vi "modify assembly.vi"(8 "error in":errorcluster, 9 "new":T1={"name"="", "Instance ID"=100, "Type"=enum."Producing", "Size (elements)"=32, "big endian?"=FALSE, "data type"=enum."Double"}, 10 "original":T1={"name"="", "Instance ID"=100, "Type"=enum."Producing", "Size (elements)"=32, "big endian?"=FALSE, "data type"=enum."Double"}, 11 "EthernetIP configuration in":refnum<class "EthernetIP configuration.lvclass">) -> (0 "error out":errorcluster, 1 "channel type/dir changed":refnum<class "EthernetIP Channel.lvclass">[](array[class]), 2 "invalidated channels":refnum<class "EthernetIP Channel.lvclass">[](array[class]), 3 "EthernetIP configuration out":refnum<class "EthernetIP configuration.lvclass">)   [LabVIEW 2013, in "EthernetIP configuration.lvclass"]
uses:
  EthernetIP configuration.lvclass
  assembly definition.ctl
  assembly type.ctl
  <vilib>/NI/Tag Bus/tag/Data Type.ctl
  channel/EthernetIP Channel.lvclass
  EthernetIP configuration.lvclass/EthernetIP configuration.ctl
  channel/EthernetIP Channel.lvclass/EthernetIP Channel.ctl
  <vilib>/NI/Tag Bus Module Framework/channel/TBM channel.lvclass/TBM channel.ctl
  <vilib>/NI/Tag Bus/tag/tag descriptor.lvclass/tag descriptor.ctl
  channel/Write Instance ID.vi
  <vilib>/NI/Tag Bus Module Framework/channel/Read channel classification.vi
  <vilib>/NI/Tag Bus Module Framework/channel/Write channel classification.vi
  channel/Read byte index.vi
  <vilib>/NI/Tag Bus/tag/read data type.vi
  <vilib>/NI/Tag Bus/tag/write data type.vi
  <vilib>/NI/Tag Bus/tag/tag descriptor.lvclass
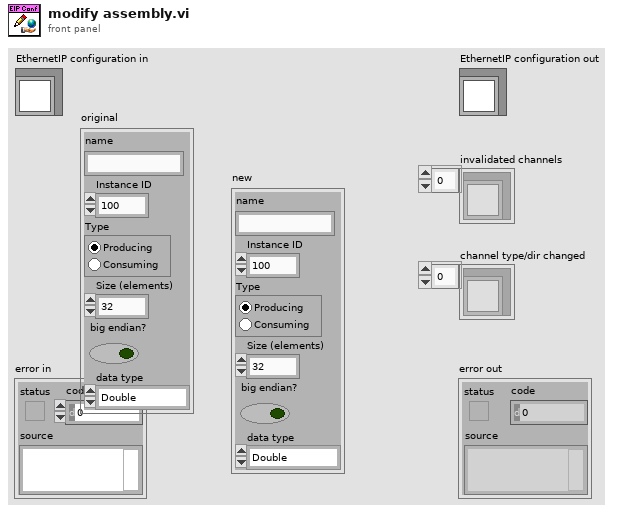
[diagram p1: front panel]
types:
  T1 = typedef "EthernetIP configuration.lvclass/assembly definition.ctl" = cluster{"name":string, "Instance ID":u32, "Type":T2, "Size (elements)":u32, "big endian?":bool, "data type":T3}
  T2 = typedef "EthernetIP configuration.lvclass/assembly type.ctl" = enum32{"Producing", "Consuming"}
  T3 = typedef "tag bus.lvlib/tag descriptor.lvclass/Data Type.ctl" = enum16{"Double", "Single", "I64", "I32", "I16", "I8", "U64", "U32", "U16", "U8", "Boolean", "String", "Array of Double", "Array of Single", "Array of I64", "Array of I32", "Array of I16", "Array of I8", "Array of U64", "Array of U32", "Array of U16", "Array of U8", "Array of Boolean", "Array of String"}
  T4 = typedef "TBM channel.lvclass/channel classification.ctl" = enum16{"input data", "output data", "processing parameter", "processing result"}
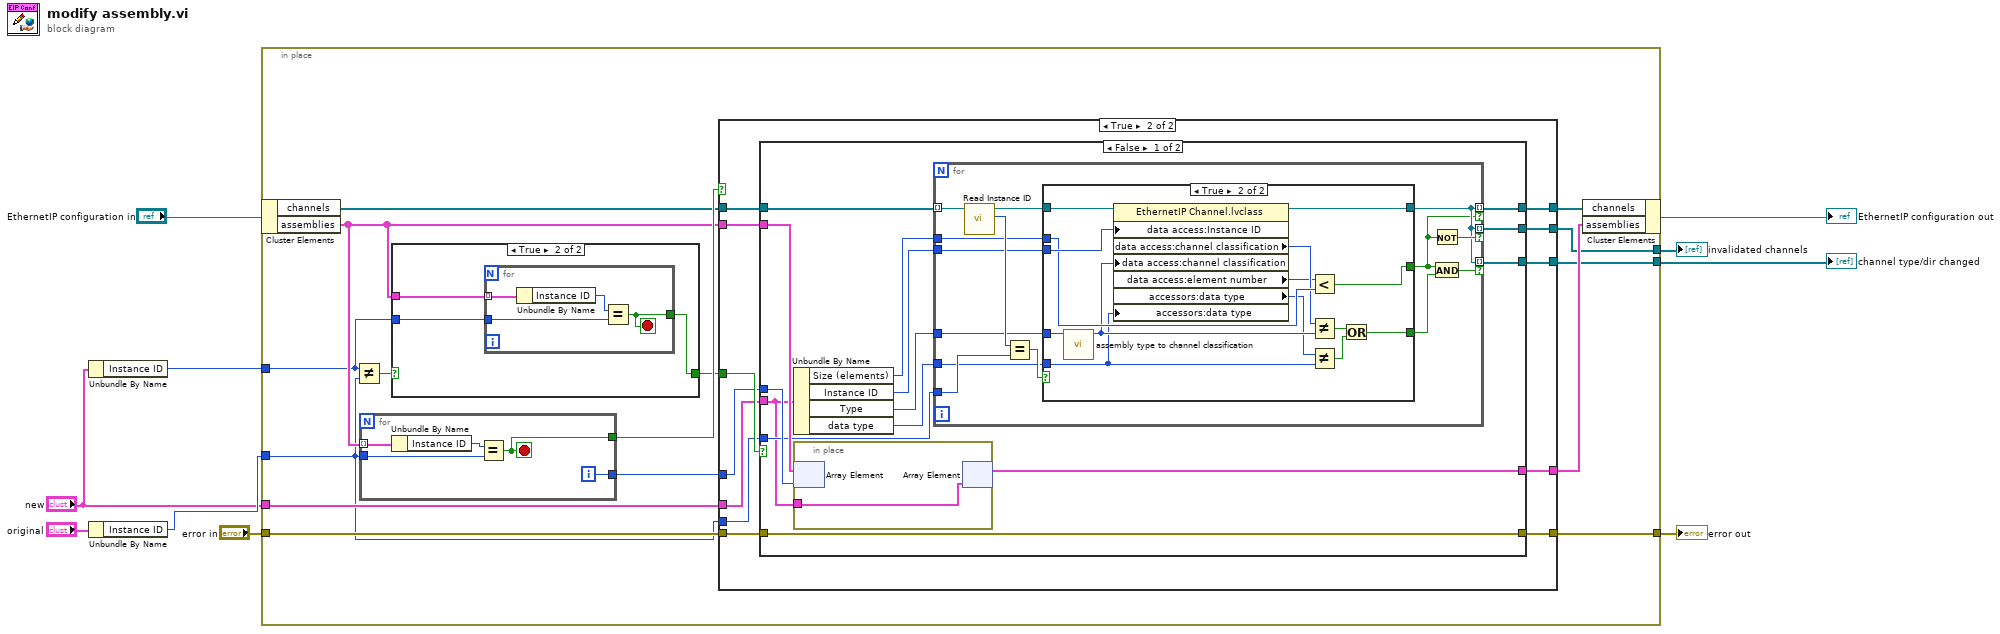
[diagram p0: block diagram]
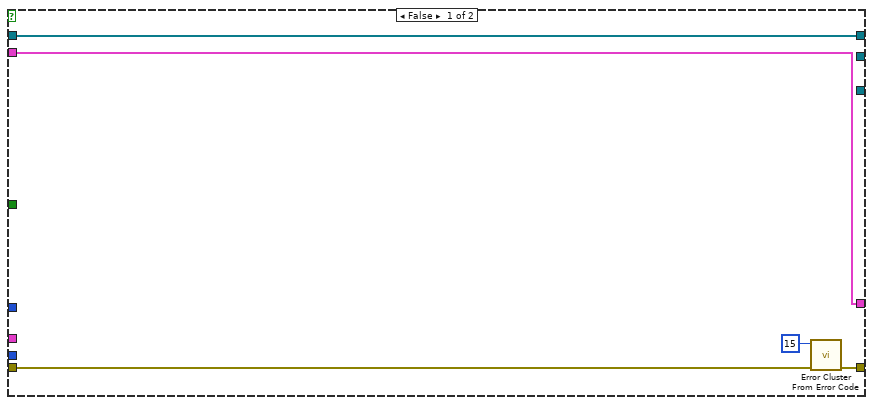
[diagram p3: hidden frame]
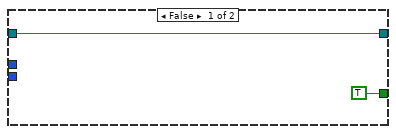
[diagram p4: hidden frame]
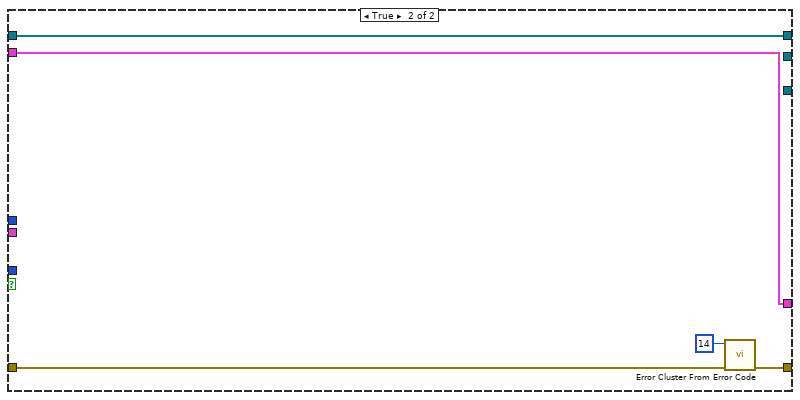
[diagram p5: hidden frame]
diagram:
  n1 = Unbundle By Name("new") -> ("Instance ID"=w6:u32)
  n2 = Unbundle By Name("original") -> ("Instance ID"=w7:u32)
  n3 = in-place {
    in-place-border: w7 -> [w14]
    in-place-border: w6 -> [w13]
    in-place-border: "error in" -> [w20]
    in-place-border: [w19] -> w4
    in-place-border: "new" -> [w16]
    in-place-border: [w15] -> w2
    in-place-border: [w11] -> w1
    n4 = in-place-cluster #1("EthernetIP configuration in") -> ("channels"=w21:refnum<class "EthernetIP Channel.lvclass">[], "assemblies"=w24:T1[])
    n5 = Not Equal?(x=w13, y=w14) -> (x != y?=w12:bool)
    n6 = for {
      tunnel: w24 -> [w105] mode=indexing
      tunnel: [w103] -> w25
      tunnel: [w102] -> w17
      tunnel: w14 -> [w101]
      i -> [w102]
      stop <- w103 stop-if-true
      n7 = Unbundle By Name(w105) -> ("Instance ID"=w104:u32)
      n8 = Equal?(x=w104, y=w101) -> (x = y?=w103:bool)
    }
    n9 = case shown="True" w12 {
      selector: w12 -> [w26 _]
      tunnel: w24 -> [_ w29]
      tunnel: [w26 w28] -> w18
      tunnel: w13 -> [_ w27]
      frame False {
      }
      frame True {
        n10 = for {
          tunnel: w29 -> [w33] mode=indexing
          tunnel: [w31] -> w28
          tunnel: w27 -> [w30]
          stop <- w31 stop-if-true
          n11 = Unbundle By Name(w33) -> ("Instance ID"=w32:u32)
          n12 = Equal?(x=w32, y=w30) -> (x = y?=w31:bool)
        }
      }
    }
    n13 = case shown="True" w25 {
      tunnel: w24 -> [w38 w44]
      tunnel: [w38 w45] -> w23
      tunnel: [w37 w46] -> w22
      tunnel: w21 -> [w37 w47]
      tunnel: w20 -> [w36 w48]
      tunnel: [w34 w49] -> w19
      tunnel: w18 -> [_ w50]
      tunnel: w17 -> [_ w43]
      tunnel: w16 -> [_ w42]
      tunnel: w14 -> [_ w41]
      tunnel: [_ w40] -> w15
      tunnel: [_ w39] -> w11
      frame False {
        n14 = call <vilib>:"Error Cluster From Error Code.vi"("error in (no error)"=w36, "error code (0)"=15) -> ("error out"=w34:errorcluster)  [unwired: 7 in]
      }
      frame True {
        n15 = case shown="False" w50 {
          tunnel: [w61 w99] -> w49
          tunnel: w48 -> [w61 w98]
          tunnel: w47 -> [w56 w97]
          tunnel: [w53 w97] -> w46
          tunnel: [w62 w96] -> w45
          tunnel: w44 -> [w64 w96]
          tunnel: w43 -> [w63 _]
          tunnel: w42 -> [w59 _]
          tunnel: w41 -> [w60 _]
          tunnel: [w57 _] -> w40
          tunnel: [w52 _] -> w39
          frame False {
            n16 = Unbundle By Name(w59) -> ("Size (elements)"=w55:u32, "Instance ID"=w58:u32, "Type"=w54:T2, "data type"=w51:T3)
            n17 = in-place {
              in-place-border: w59 -> [w95]
              n18 = in-place-array #2(w64, w63) -> ()  [unwired: 1 out]
              n19 = in-place-array #2(w95) -> (w62:T1[])  [unwired: 1 out]
            }
            n20 = for {
              tunnel: w56 -> [w78] mode=indexing
              tunnel: w60 -> [w76]
              tunnel: [w69] -> w53 mode=indexing if=w68
              tunnel: w58 -> [w73]
              tunnel: [w69] -> w57 mode=indexing if=w72
              tunnel: w55 -> [w71]
              tunnel: w54 -> [w70]
              tunnel: [w69] -> w52 mode=indexing if=w66
              tunnel: w51 -> [w65]
              n21 = call "Read Instance ID.vi"("EthernetIP Channel in"=w78) -> ("Instance ID"=w77:u32, "EthernetIP Channel out"=w75:refnum<class "EthernetIP Channel.lvclass">)  [unwired: 8 in, 1 out]
              n22 = Equal?(x=w77, y=w76) -> (x = y?=w74:bool)
              n23 = case shown="True" w74 {
                tunnel: w75 -> [w79 w94]
                tunnel: [w79 w93] -> w69
                tunnel: w73 -> [_ w92]
                tunnel: [TRUE w90] -> w68
                tunnel: w71 -> [_ w91]
                tunnel: w70 -> [_ w89]
                tunnel: [_ w82] -> w67
                tunnel: w65 -> [_ w83]
                frame False {
                }
                frame True {
                  n24 = call "assembly type to channel classification.vi"("Type"=w89) -> ("channel classification"=w87:T4)  [unwired: 10 in]
                  n25 = property class="EthernetIP Channel.lvclass"(reference=w94, "data access:Instance ID"=w92, "data access:channel classification"=w87, "accessors:data type"=w83) -> (reference out=w93:refnum<class "EthernetIP Channel.lvclass">, "data access:channel classification"=w88:T4, "data access:element number"=w85:i32, "accessors:data type"=w84:T3)  [unwired: 1 in, 1 out]
                  n26 = Less?(x=w85, y=w91) -> (x < y?=w90:bool)
                  n27 = Not Equal?(x=w88, y=w87) -> (x != y?=w86:bool)
                  n28 = Not Equal?(x=w84, y=w83) -> (x != y?=w81:bool)
                  n29 = Or(x=w86, y=w81) -> (x .or. y?=w82:bool)
                }
              }
              n30 = Not(x=w68) -> (.not. x?=w72:bool)
              n31 = And(x=w68, y=w67) -> (x .and. y?=w66:bool)
            }
          }
          frame True {
            n32 = call <vilib>:"Error Cluster From Error Code.vi"("error in (no error)"=w98, "error code (0)"=14) -> ("error out"=w99:errorcluster)  [unwired: 7 in]
          }
        }
      }
    }
    n33 = in-place-cluster #1("channels"=w22, "assemblies"=w23) -> (→"EthernetIP configuration out":refnum<class "EthernetIP configuration.lvclass">)
  }
  "error out" <- w4
  "invalidated channels" <- w2
  "channel type/dir changed" <- w1
